vi "Decrease Dimension.vi"(11 "2D Array IN":u64[][](array[numeric])=[[12, 11, 34, 2, 45], [34, 3, 4, 5, 6], [45, 7, 8, 9, 10], [11, 12, 13, 43, 33], [22, 15, 16, 17, 18], [47, 21, 22, 23, 34], [35, 24, 25, 26, 27], [25, 31, 32, 33, 35], [33, 41, 42, 43, 44], [7, 8, 9, 17, 23]]) -> (3 "Digit Out":u64)   [LabVIEW 2023]
panel:
  out "1D Array Out":u64[](array[numeric])
  # "Намалява размерността на 2D масив до 1D такъв или до число."
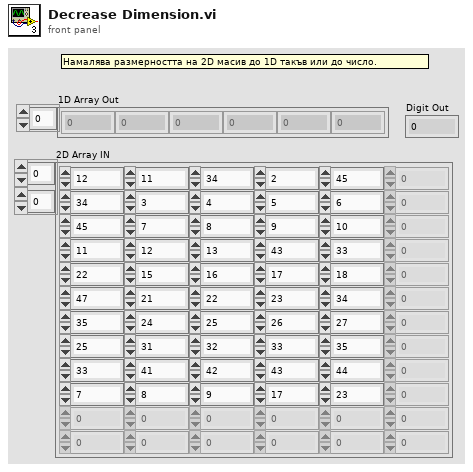
[diagram p1: front panel]
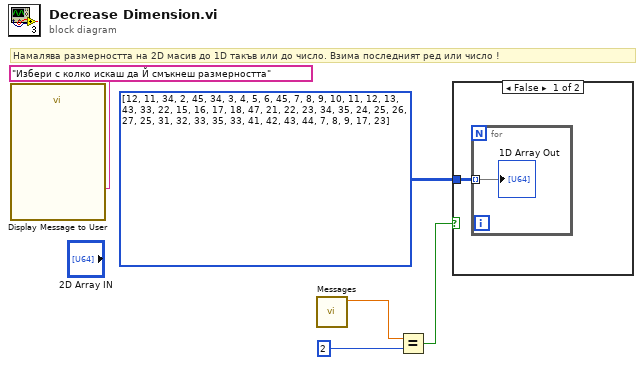
[diagram p0: block diagram]
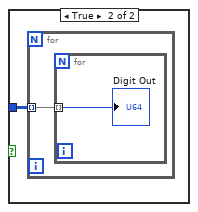
[diagram p2: hidden frame]
diagram:
  # "Намалява размерността на 2D масив до 1D такъв или до число. Взима последният ред или число !"
  n1 = call "Display Message to User"("Message"="Избери с колко искаш да Й смъкнеш размерността") -> ()  [unwired: 9 in, 2 out]
  n2 = call "Messages.vi"() -> (";)   ?"=w4:dbl)  [unwired: 11 in]
  n3 = Equal?(x=w4, y=u64 2) -> (x = y?=w2:bool)
  n4 = case shown="False" w2 {
    tunnel: u64[][] [[12, 11, 34, 2, 45], [34, 3, 4, 5, 6], [45, 7, 8, 9, 10], [11, 12, 13, 43, 33], [22, 15, 16, 17, 18], [47, 21, 22, 23, 34], [35, 24, 25, 26, 27], [25, 31, 32, 33, 35], [33, 41, 42, 43, 44], [7, 8, 9, 17, 23]] ("2D Array") -> [w6 w8]
    frame False {
      n5 = for {
        tunnel: w6 -> [w7] mode=indexing
        "1D Array Out" <- w7
      }
    }
    frame True {
      n6 = for {
        tunnel: w8 -> [w9] mode=indexing
        n7 = for {
          tunnel: w9 -> [w10] mode=indexing
          "Digit Out" <- w10
        }
      }
    }
  }
